vi "Pcre2JitStackAssign8.vi"(8 "error in":errorcluster, 11 "pJitStack":u64 format="%.0x") -> (0 "error out":errorcluster, 3 "pMatchContext":u64 format="%.0x")   [LabVIEW 2021, in "libpcre2-8.lvlib"]
uses:
  libpcre2-8.lvlib
  libpcre2-8-x32.dll
panel:
  in  "pMatchContext":u64 format="%.0x"
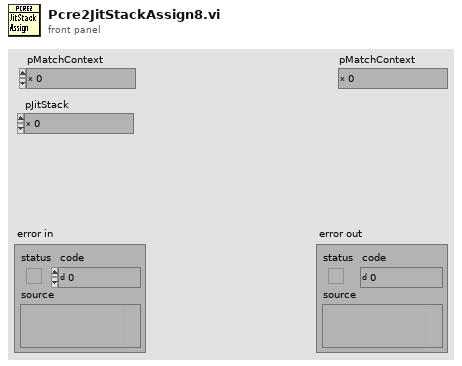
[diagram p1: front panel]
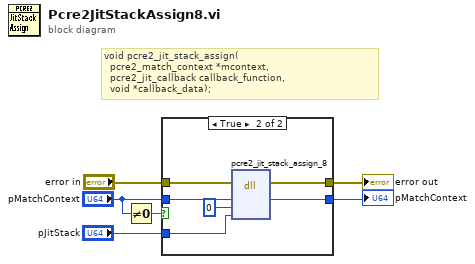
[diagram p0: block diagram]
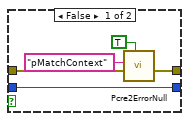
[diagram p2: hidden frame]
diagram:
  # "void pcre2_jit_stack_assign(\n  pcre2_match_context *mcontext,\n  pcre2_jit_callback callback_function,\n  void *callback_data);"
  n1 = Not Equal To 0?(x="pMatchContext") -> (x != 0?=w1:bool)
  n2 = case shown="True" w1 {
    tunnel: "error in" -> [w10 w17]
    tunnel: "pMatchContext" -> [w7 w16]
    tunnel: [w7 w15] -> w4
    tunnel: [w11 w13] -> w3
    tunnel: "pJitStack" -> [_ w12]
    frame False {
      n3 = call "Pcre2ErrorNull.vi"("IsPointer? (F)"=TRUE, "error in"=w10, "What"="pMatchContext") -> ("error out"=w11:errorcluster)  [unwired: 8 in]
    }
    frame True {
      n4 = dll-call lib="libpcre2-8-x*.dll" fn="pcre2_jit_stack_assign_8"(error in=w17, "mcontext"=w16, "callback_function"=u64 0, "callback_data"=w12) -> (error out=w13:errorcluster, "mcontext"=w15:u64)  [unwired: 5 in, 1 out]
    }
  }
  "error out" <- w3
  "pMatchContext" <- w4
